vi "generate knight neighbours--trigonometric order.vi"(1 "current square (chessboard_index)":T1) -> (0 "neighbours (chessboard_index)":T1[](array[typedef]))   [LabVIEW 2020, in "core.lvlib"]
uses:
  core.lvlib
  core_data/chessboard_index.ctl
  core_data/core_data.lvlib
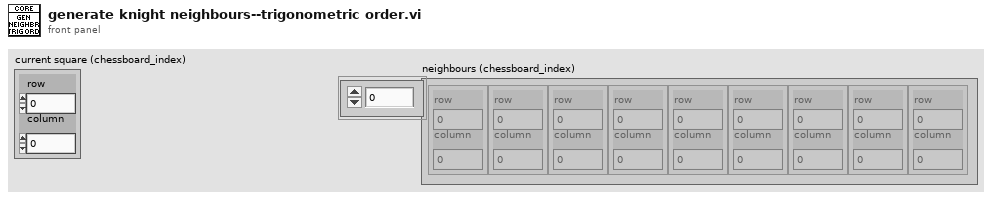
[diagram p1: front panel]
types:
  T1 = typedef "core.lvlib/core_data.lvlib/chessboard_index.ctl" = cluster{"row":u8, "column":u8}
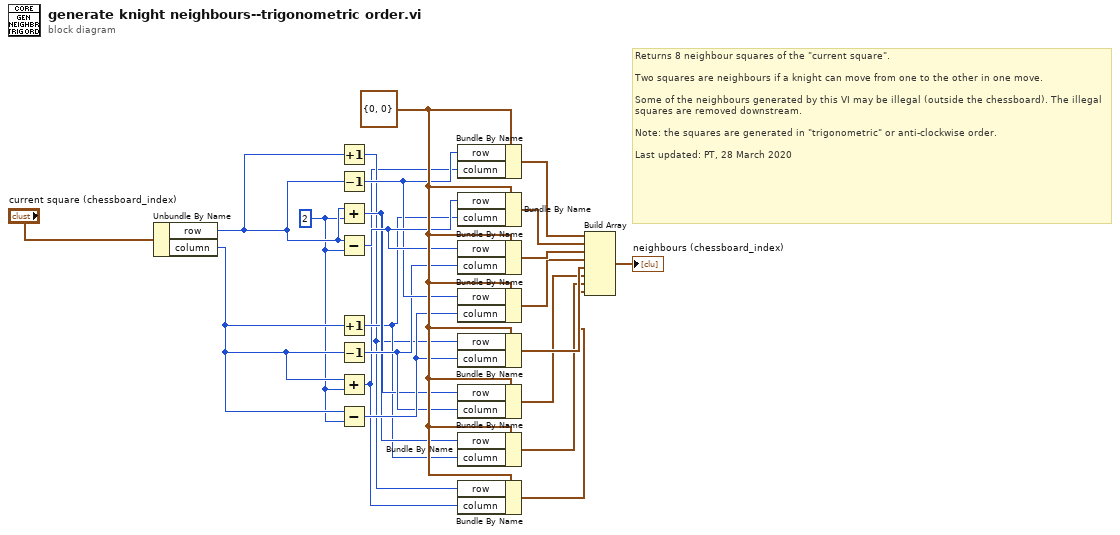
[diagram p0: block diagram]
diagram:
  w18 = T1 {"row"=0, "column"=0} ("2D array location 2")
  w19 = u8 2 ("y")
  # "Returns 8 neighbour squares of the \"current square\".\n\nTwo squares are neighbours if a knight can move from one to the other in one move. \n\nSome of the neighbours generated by this VI may be illegal (outside the chessboard). The illegal squares are removed downstream.\n\nNote: the squares are generated in \"trigonometric\" or anti-clockwise order.\n\nLast updated: PT, 28 March 2020"
  n1 = Unbundle By Name("current square (chessboard_index)") -> ("row"=w21:u8, "column"=w20:u8)
  n2 = Increment(x=w21) -> (x+1=w2:u8)
  n3 = Decrement(x=w21) -> (x-1=w7:u8)
  n4 = Add(x=w21, y=w19) -> (x+y=w4:u8)
  n5 = Subtract(x=w21, y=w19) -> (x-y=w8:u8)
  n6 = Increment(x=w20) -> (x+1=w3:u8)
  n7 = Decrement(x=w20) -> (x-1=w5:u8)
  n8 = Add(x=w20, y=w19) -> (x+y=w1:u8)
  n9 = Subtract(x=w20, y=w19) -> (x-y=w6:u8)
  n10 = Bundle By Name(cluster=w18, "row"=w7, "column"=w1) -> (w17:T1)
  n11 = Bundle By Name(cluster=w18, "row"=w8, "column"=w3) -> (w16:T1)
  n12 = Bundle By Name(cluster=w18, "row"=w8, "column"=w5) -> (w15:T1)
  n13 = Bundle By Name(cluster=w18, "row"=w7, "column"=w6) -> (w14:T1)
  n14 = Bundle By Name(cluster=w18, "row"=w2, "column"=w6) -> (w13:T1)
  n15 = Bundle By Name(cluster=w18, "row"=w4, "column"=w5) -> (w12:T1)
  n16 = Bundle By Name(cluster=w18, "row"=w4, "column"=w3) -> (w11:T1)
  n17 = Bundle By Name(cluster=w18, "row"=w2, "column"=w1) -> (w10:T1)
  n18 = Build Array(w17, w16, w15, w14, w13, w12, w11, w10) -> (→"neighbours (chessboard_index)":T1[])
